vi "Read Configuration Parameters.vi"(8 "error in (no error)":errorcluster, 10 "refnum":T1, 11 "Example Configuration Dialog in":refnum<class "Example Configuration Dialog.lvclass">) -> (0 "error out":errorcluster, 2 "refnum out":T1, 3 "Example Configuration Dialog out":refnum<class "Example Configuration Dialog.lvclass">)   [LabVIEW 2020, in "Example Configuration Dialog.lvlib" / "Example Configuration Dialog.lvclass"]
uses:
  Example Configuration Dialog.lvclass
  <vilib>/Utility/config.llb/Config Data RefNum.ctl
  Example Configuration Dialog.lvclass/Example Configuration Dialog.ctl
  <vilib>/Utility/config.llb/Read Key (I32).vi
  <vilib>/Utility/config.llb/Read Key (String).vi
  Configuration.lvclass
  <vilib>/Utility/config.llb/NI_LVConfig.lvlib
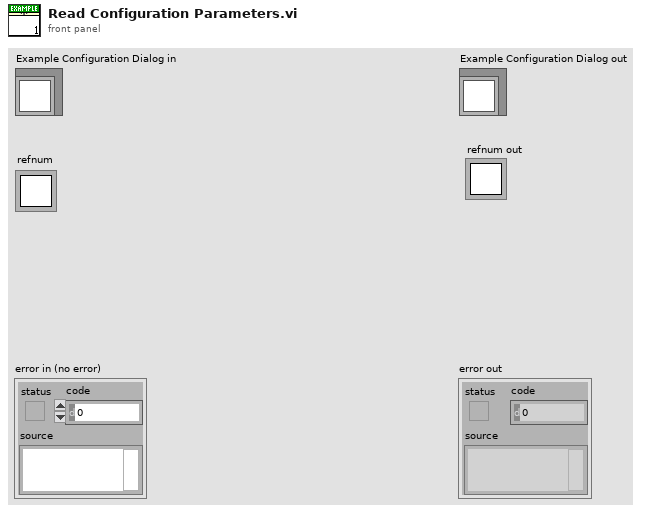
[diagram p1: front panel]
types:
  T1 = typedef "NI_LVConfig.lvlib/Config Data RefNum.ctl" = refnum<k1>
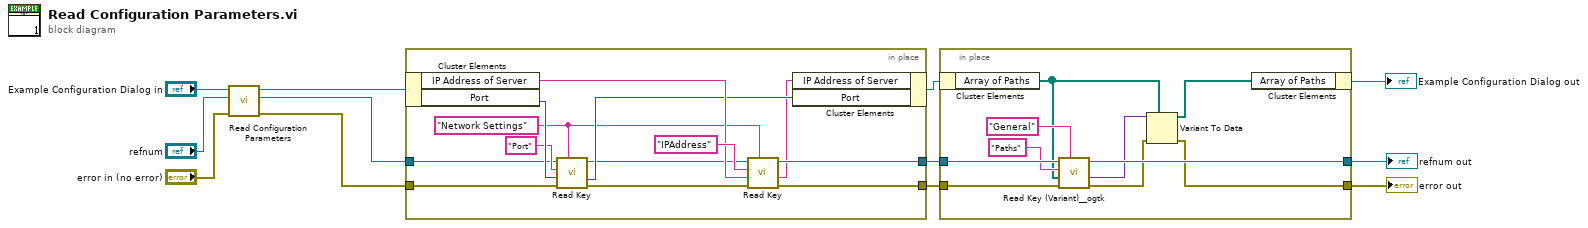
[diagram p0: block diagram]
diagram:
  n1 = call-parent "Read Configuration Parameters.vi"("error in (no error)"="error in (no error)", "refnum"="refnum", "Configuration in"="Example Configuration Dialog in") -> ("error out"=w8:errorcluster, "refnum out"=w9:T1, "Configuration out"=w7:refnum<class "Example Configuration Dialog.lvclass">)  [unwired: 6 in]
  n2 = in-place "In Place Element Structure" {
    in-place-border: w9 -> [w15]
    in-place-border: w8 -> [w21]
    in-place-border: [w23] -> w4
    in-place-border: [w22] -> w5
    w17 = "Network Settings" ("section")
    n3 = in-place-cluster #1(w7) -> ("IP Address of Server"=w24:string, "Port"=w19:i32)
    n4 = call-poly <vilib>:"Read Key.vi"("section"=w17, "error in (no error)"=w21, "default value"=w19, "key"="Port", "refnum"=w15) -> ("error out"=w20:errorcluster, "value"=w18:i32, "refnum out"=w14:T1)  [unwired: 3 in, 1 out]
    n5 = call-poly <vilib>:"Read Key.vi"("section"=w17, "error in (no error)"=w20, "default value"=w24, "key"="IPAddress", "refnum"=w14) -> ("error out"=w23:errorcluster, "value"=w13:string, "refnum out"=w22:T1)  [unwired: 3 in, 1 out]
    n6 = in-place-cluster #1("IP Address of Server"=w13, "Port"=w18) -> (w6:refnum<class "Example Configuration Dialog.lvclass">)
  }
  n7 = in-place "In Place Element Structure" {
    in-place-border: w5 -> [w35]
    in-place-border: w4 -> [w34]
    in-place-border: [w26] -> w3
    in-place-border: [w31] -> w2
    n8 = in-place-cluster #2(w6) -> ("Array of Paths"=w30:path[])
    n9 = call <userlib>:"Read Key (Variant)__ogtk.vi"("section"="General", "error in (no error)"=w34, "type"=w30, "key (optional)"="Paths", "refnum"=w35) -> ("error out"=w27:errorcluster, "key-value"=w29:variant, "refnum out"=w31:T1)  [unwired: 3 in, 1 out]
    n10 = Variant To Data(error in=w27, type=w30, Variant=w29) -> (data=w28:path[], error out=w26:errorcluster)
    n11 = in-place-cluster #2("Array of Paths"=w28) -> (→"Example Configuration Dialog out":refnum<class "Example Configuration Dialog.lvclass">)
  }
  "error out" <- w3
  "refnum out" <- w2
